vi "Servo MSMT SpecAn Set DC Params.vi"(8 "error in (no error)":errorcluster, 10 "Step In":refnum<k7>, 11 "Servo MSMT in":refnum<class "Servo MSMT.lvclass">) -> (0 "error out":errorcluster, 2 "Step Out":refnum<k7>, 3 "Servo MSMT out":refnum<class "Servo MSMT.lvclass">)   [LabVIEW 2018, in "Servo MSMT.lvlib" / "Servo MSMT.lvclass"]
uses:
  Servo MSMT.lvclass
  Servo MSMT.lvclass/Servo MSMT.ctl
  Protected Methods/Read DC Pins.vi
  Protected Methods/Read PAE Pins.vi
  Protected Methods/Read PAE Enable Override_.vi
  Plugins/TestStand API Tools (TSAT).lvlibp/Step Actions/TSAT Step Actions.lvlib
  Plugins/Measurement Interface.lvlibp/Measurement Interface.lvclass
  C:/Sequence Automation/Plugins/Measurement Interface.lvlibp/Measurement Interface.lvclass
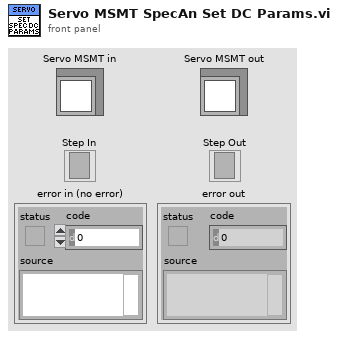
[diagram p1: front panel]
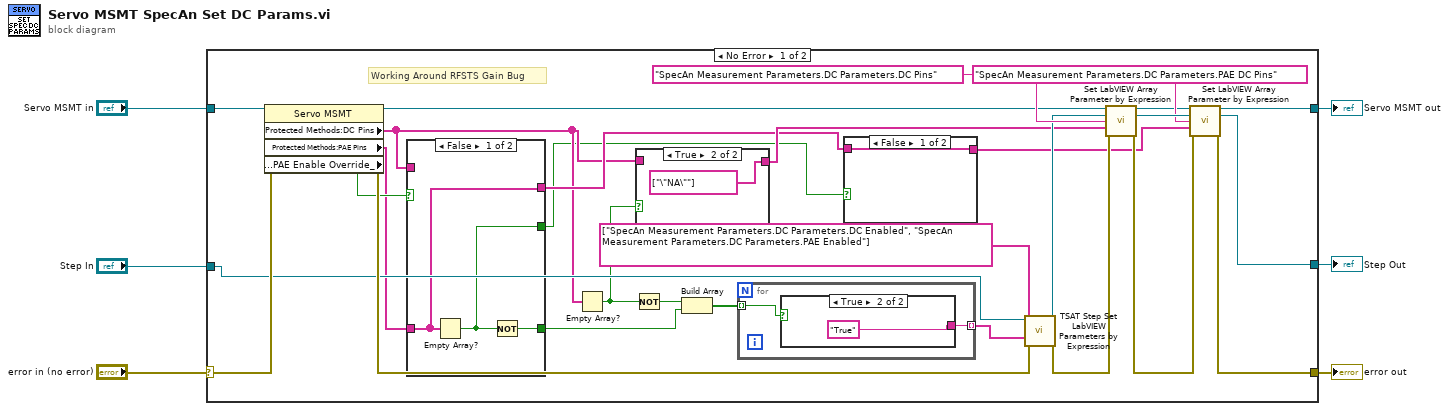
[diagram p0: block diagram]
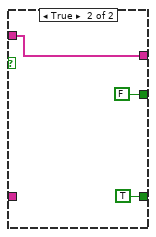
[diagram p2: hidden frame]
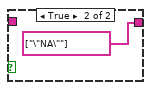
[diagram p3: hidden frame]
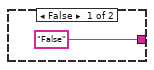
[diagram p5: hidden frame]
diagram:
  n1 = case shown="No Error" "error in (no error)" {
    selector: "error in (no error)" -> [w34 w51]
    tunnel: [w30 w51] -> w5
    tunnel: [w24 w50] -> w3
    tunnel: "Servo MSMT in" -> [w33 w50]
    tunnel: "Step In" -> [w21 w49]
    tunnel: [w28 w49] -> w1
    frame No Error {
      # "Working Around RFSTS Gain Bug"
      n2 = property class="Servo MSMT"(reference=w33, error in=w34) -> (reference out=w26:refnum<class "Servo MSMT.lvclass">, error out=w23:errorcluster, "Protected Methods:DC Pins"=w8:string[], "Protected Methods:PAE Pins"=w11:string[], "Protected Methods:PAE Enable Override_"=w12:bool)
      n3 = case shown="False" w12 {
        tunnel: w11 -> [w37 _]
        tunnel: [w36 TRUE] -> w10
        tunnel: [w37 w39] -> w9
        tunnel: w8 -> [_ w39]
        tunnel: [w35 FALSE] -> w7
        frame False {
          n4 = Empty Array?(array=w37) -> (empty?=w35:bool)
          n5 = Not(x=w35) -> (.not. x?=w36:bool)
        }
        frame True {
        }
      }
      n6 = Empty Array?(array=w8) -> (empty?=w16:bool)
      n7 = Not(x=w16) -> (.not. x?=w13:bool)
      n8 = case shown="True" w16 {
        tunnel: w8 -> [w43 _]
        tunnel: [w43 string[] ["\"NA\""] ("Protected Methods:DC Pins")] -> w15
        frame False {
        }
        frame True {
        }
      }
      n9 = Build Array(w13, w10) -> (w19:bool[])
      n10 = for {
        tunnel: w19 -> [w46] mode=indexing
        tunnel: [w45] -> w18 mode=indexing
        n11 = case shown="True" w46 {
          tunnel: ["False" "True"] -> w45
          frame False {
          }
          frame True {
          }
        }
      }
      n12 = case shown="False" w7 {
        tunnel: w9 -> [w41 _]
        tunnel: [w41 string[] ["\"NA\""] ("Protected Methods:DC Pins")] -> w14
        frame False {
        }
        frame True {
        }
      }
      n13 = call "TSAT Step Set LabVIEW Parameters by Expression.vi"("Error In"=w23, "Value Expressions"=w18, "Parameters to Set"=string[] ["SpecAn Measurement Parameters.DC Parameters.DC Enabled", "SpecAn Measurement Parameters.DC Parameters.PAE Enabled"], "Step In"=w21) -> ("Error Out"=w22:errorcluster, "Step Out"=w20:refnum<k7>)  [unwired: 6 in]
      n14 = call "Set LabVIEW Array Parameter by Expression.vi"("Measurement Interface in"=w26, "Step In"=w20, "LabVIEW Parameter to Set"="SpecAn Measurement Parameters.DC Parameters.DC Pins", "Array of Expresssions"=w15, "error in (no error)"=w22) -> ("Measurement Interface out"=w25:refnum<class "Servo MSMT.lvclass">, "Step Out"=w29:refnum<k7>, "error out"=w31:errorcluster)  [unwired: 8 in]
      n15 = call "Set LabVIEW Array Parameter by Expression.vi"("Measurement Interface in"=w25, "Step In"=w29, "LabVIEW Parameter to Set"="SpecAn Measurement Parameters.DC Parameters.PAE DC Pins", "Array of Expresssions"=w14, "error in (no error)"=w31) -> ("Measurement Interface out"=w24:refnum<class "Servo MSMT.lvclass">, "Step Out"=w28:refnum<k7>, "error out"=w30:errorcluster)  [unwired: 8 in]
    }
    frame Error {
    }
  }
  "error out" <- w5
  "Servo MSMT out" <- w3
  "Step Out" <- w1
